vi "Trigger Circuitry.vi"(6 "State Machine State":T2, 7 "Trigger Type":T3(ring)=enum."Software Trigger", 9 "Analog Trigger Setup":T1, 10 "Digital Line Read":bool, 11 "Software Trigger from Host":bool) -> (0 "Trigger Info":cluster{"Trigger":bool, "Trig Offset":u8}, 2 "Trigger Out":bool, 3 "Analog Arm Trig":bool)   [LabVIEW 2011]
uses:
  <instrlib>/FlexRIO/Libraries/Acquisition Engine/FPGA/Interface/acqEngineStates v1.ctl
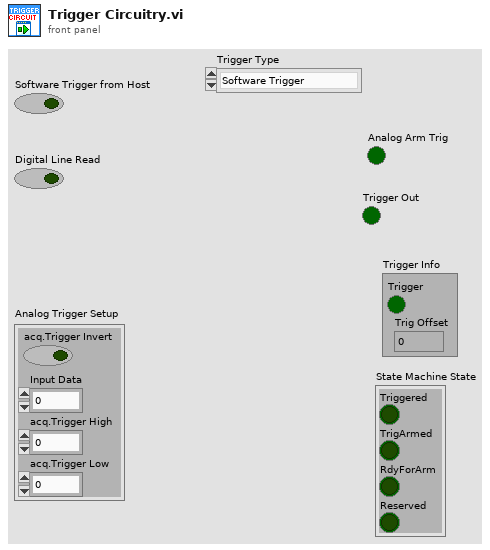
[diagram p1: front panel]
types:
  T1 = cluster{"acq.Trigger Invert":bool, "Input Data":i16, "acq.Trigger High":i16, "acq.Trigger Low":i16}
  T2 = typedef "acqEngineStates v1.ctl" = cluster{"Triggered":bool, "TrigArmed":bool, "RdyForArm":bool, "Reserved":bool}
  T3 = enum8{"Immediate Trigger", "Software Trigger", "External Digital Trigger", "Analog Trigger"}
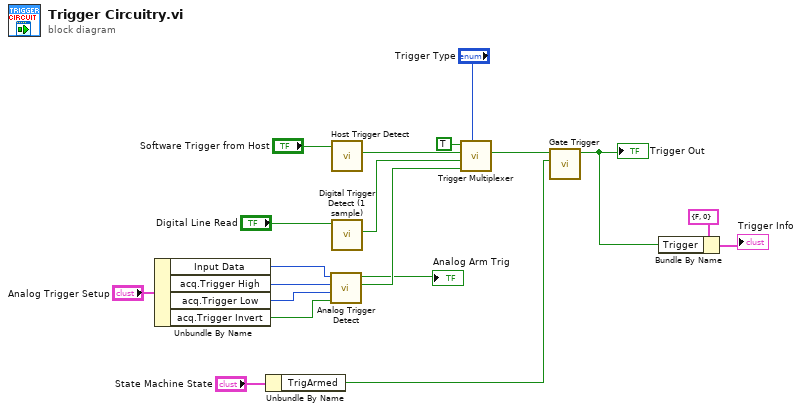
[diagram p0: block diagram]
diagram:
  n1 = Unbundle By Name("Analog Trigger Setup") -> ("Input Data"=w8:i16, "acq.Trigger High"=w7:i16, "acq.Trigger Low"=w6:i16, "acq.Trigger Invert"=w5:bool)
  n2 = Unbundle By Name("State Machine State") -> ("TrigArmed"=w11:bool)
  n3 = call <userlib>:"Analog Trigger Detect.vi"("acq.Trigger Invert"=w5, "acq.Trigger High"=w6, "acq.Trigger Low"=w7, "Input Data"=w8) -> ("Analog Trigger Detect"=w15:bool, "Analog Arm Trig"=→"Analog Arm Trig":bool)  [unwired: 6 in]
  n4 = call <userlib>:"Host Trigger Detect.vi"("Software Trigger from Host"="Software Trigger from Host") -> ("Host Rising Edge Detect"=w17:bool)  [unwired: 10 in]
  n5 = call <userlib>:"Digital Trigger Detect (1 sample).vi"("Digital Line Read"="Digital Line Read") -> ("Rising Edge"=w16:bool)  [unwired: 9 in, 1 out]
  n6 = call <userlib>:"Trigger Multiplexer.vi"("Trigger Type"="Trigger Type", "Analog Trigger"=w15, "Digital Trigger"=w16, "Software Trigger"=w17, "Immediate Trigger"=TRUE) -> ("Trigger Out"=w12:bool)  [unwired: 6 in]
  n7 = call <userlib>:"Gate Trigger.vi"("Gate Signal'"=w11, "Trigger"=w12) -> ("Ref Trig"=w1:bool)  [unwired: 9 in]
  "Trigger Out" <- w1
  n8 = Bundle By Name(cluster=cluster{"Trigger":bool, "Trig Offset":u8} {"Trigger"=FALSE, "Trig Offset"=0} ("Trigger Info"), "Trigger"=w1) -> (→"Trigger Info":cluster{"Trigger":bool, "Trig Offset":u8})
